vi "test-transform2d.vi"(8 "error in (no error)":errorcluster) -> (0 "error out":errorcluster, 3 "All PASSED":bool)   [LabVIEW 2019]
uses:
  <vilib>/Rock Robotics/WPI/ThirdParty/JAS_Junk/TrajLib/Transform2d_Create_PosePose.vi
  <vilib>/Rock Robotics/WPI/ThirdParty/JAS_Junk/TrajLib/Pose2d_New.vi
  <vilib>/Rock Robotics/WPI/ThirdParty/JAS_Junk/TrajLib/Pose2d_TransformBy.vi
  <vilib>/Rock Robotics/WPI/ThirdParty/JAS_Junk/TrajLib/Translation2d_Equals.vi
  <vilib>/Rock Robotics/WPI/ThirdParty/JAS_Junk/TrajLib/Rotation2d_Equals.vi
  <vilib>/Rock Robotics/WPI/ThirdParty/JAS_Junk/TrajLib/Translation2d_UnaryMinus.vi
  <vilib>/Rock Robotics/WPI/ThirdParty/JAS_Junk/TrajLib/Rotation2d_UnaryMinus.vi
  <vilib>/Rock Robotics/WPI/ThirdParty/JAS_Junk/TrajLib/Translation2d_RotateBy.vi
  <vilib>/Rock Robotics/WPI/ThirdParty/JAS_Junk/TrajLib/Translation2d_Minus.vi
  <vilib>/Rock Robotics/WPI/ThirdParty/JAS_Junk/TrajLib/Rotation2d_Minus.vi
  <vilib>/Rock Robotics/WPI/ThirdParty/JAS_Junk/TrajLib/Translation2d_Plus.vi
  <vilib>/Rock Robotics/WPI/ThirdParty/JAS_Junk/TrajLib/Rotation2d_Plus.vi
  <vilib>/Rock Robotics/WPI/ThirdParty/JAS_Junk/TrajLib/Util_CalcDist.vi
  <vilib>/Rock Robotics/WPI/ThirdParty/JAS_Junk/TrajLib/Rotation2d_RotateBy.vi
  <vilib>/Rock Robotics/WPI/ThirdParty/JAS_Junk/TrajLib/Rotation2d_CreateXY.vi
  <vilib>/Rock Robotics/WPI/ThirdParty/JAS_Junk/TrajLib/Trajectory_Library.lvlib
panel:
  out "Test 2 Passed":bool
  out "T1 Passed":bool
  out "T5 - ANG = 43 Deg":dbl
  out "T5 - Y2 = 4.4":dbl
  out "T5 - X2= -3.33":dbl
  out "T5 - Y = 4.4":dbl
  out "T5 - X = -3.33":dbl
  # "Transform2D Test  --- NOT DONE"
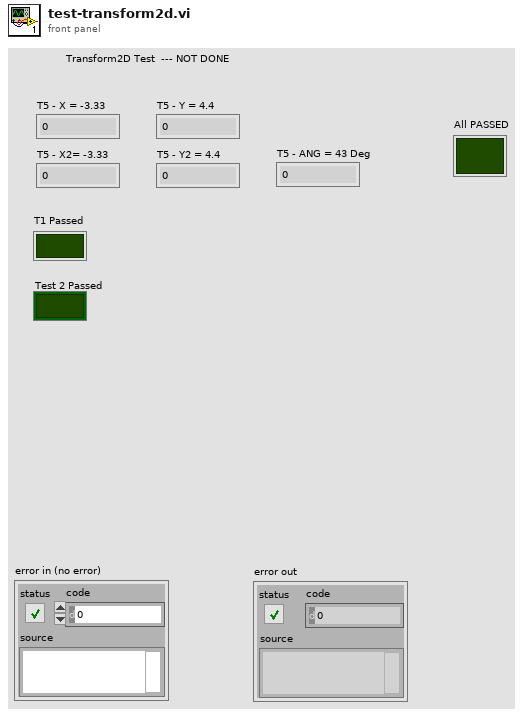
[diagram p1: front panel]
types:
  T1 = typedef "Trajectory_Library.lvlib/TRANSLATION2D.ctl" = cluster{"X":dbl, "Y":dbl}
  T2 = typedef "Trajectory_Library.lvlib/ROTATION2D.ctl" = cluster{"VALUE":dbl, "COS":dbl, "SIN":dbl}
  T3 = typedef "Trajectory_Library.lvlib/TRANSFORM2D.ctl" = cluster{"TRANSLATION":T1, "ROTATION":T2}
  T4 = typedef "Trajectory_Library.lvlib/POSE2D.ctl" = cluster{"TRANSLATION":T1, "ROTATION":T2}
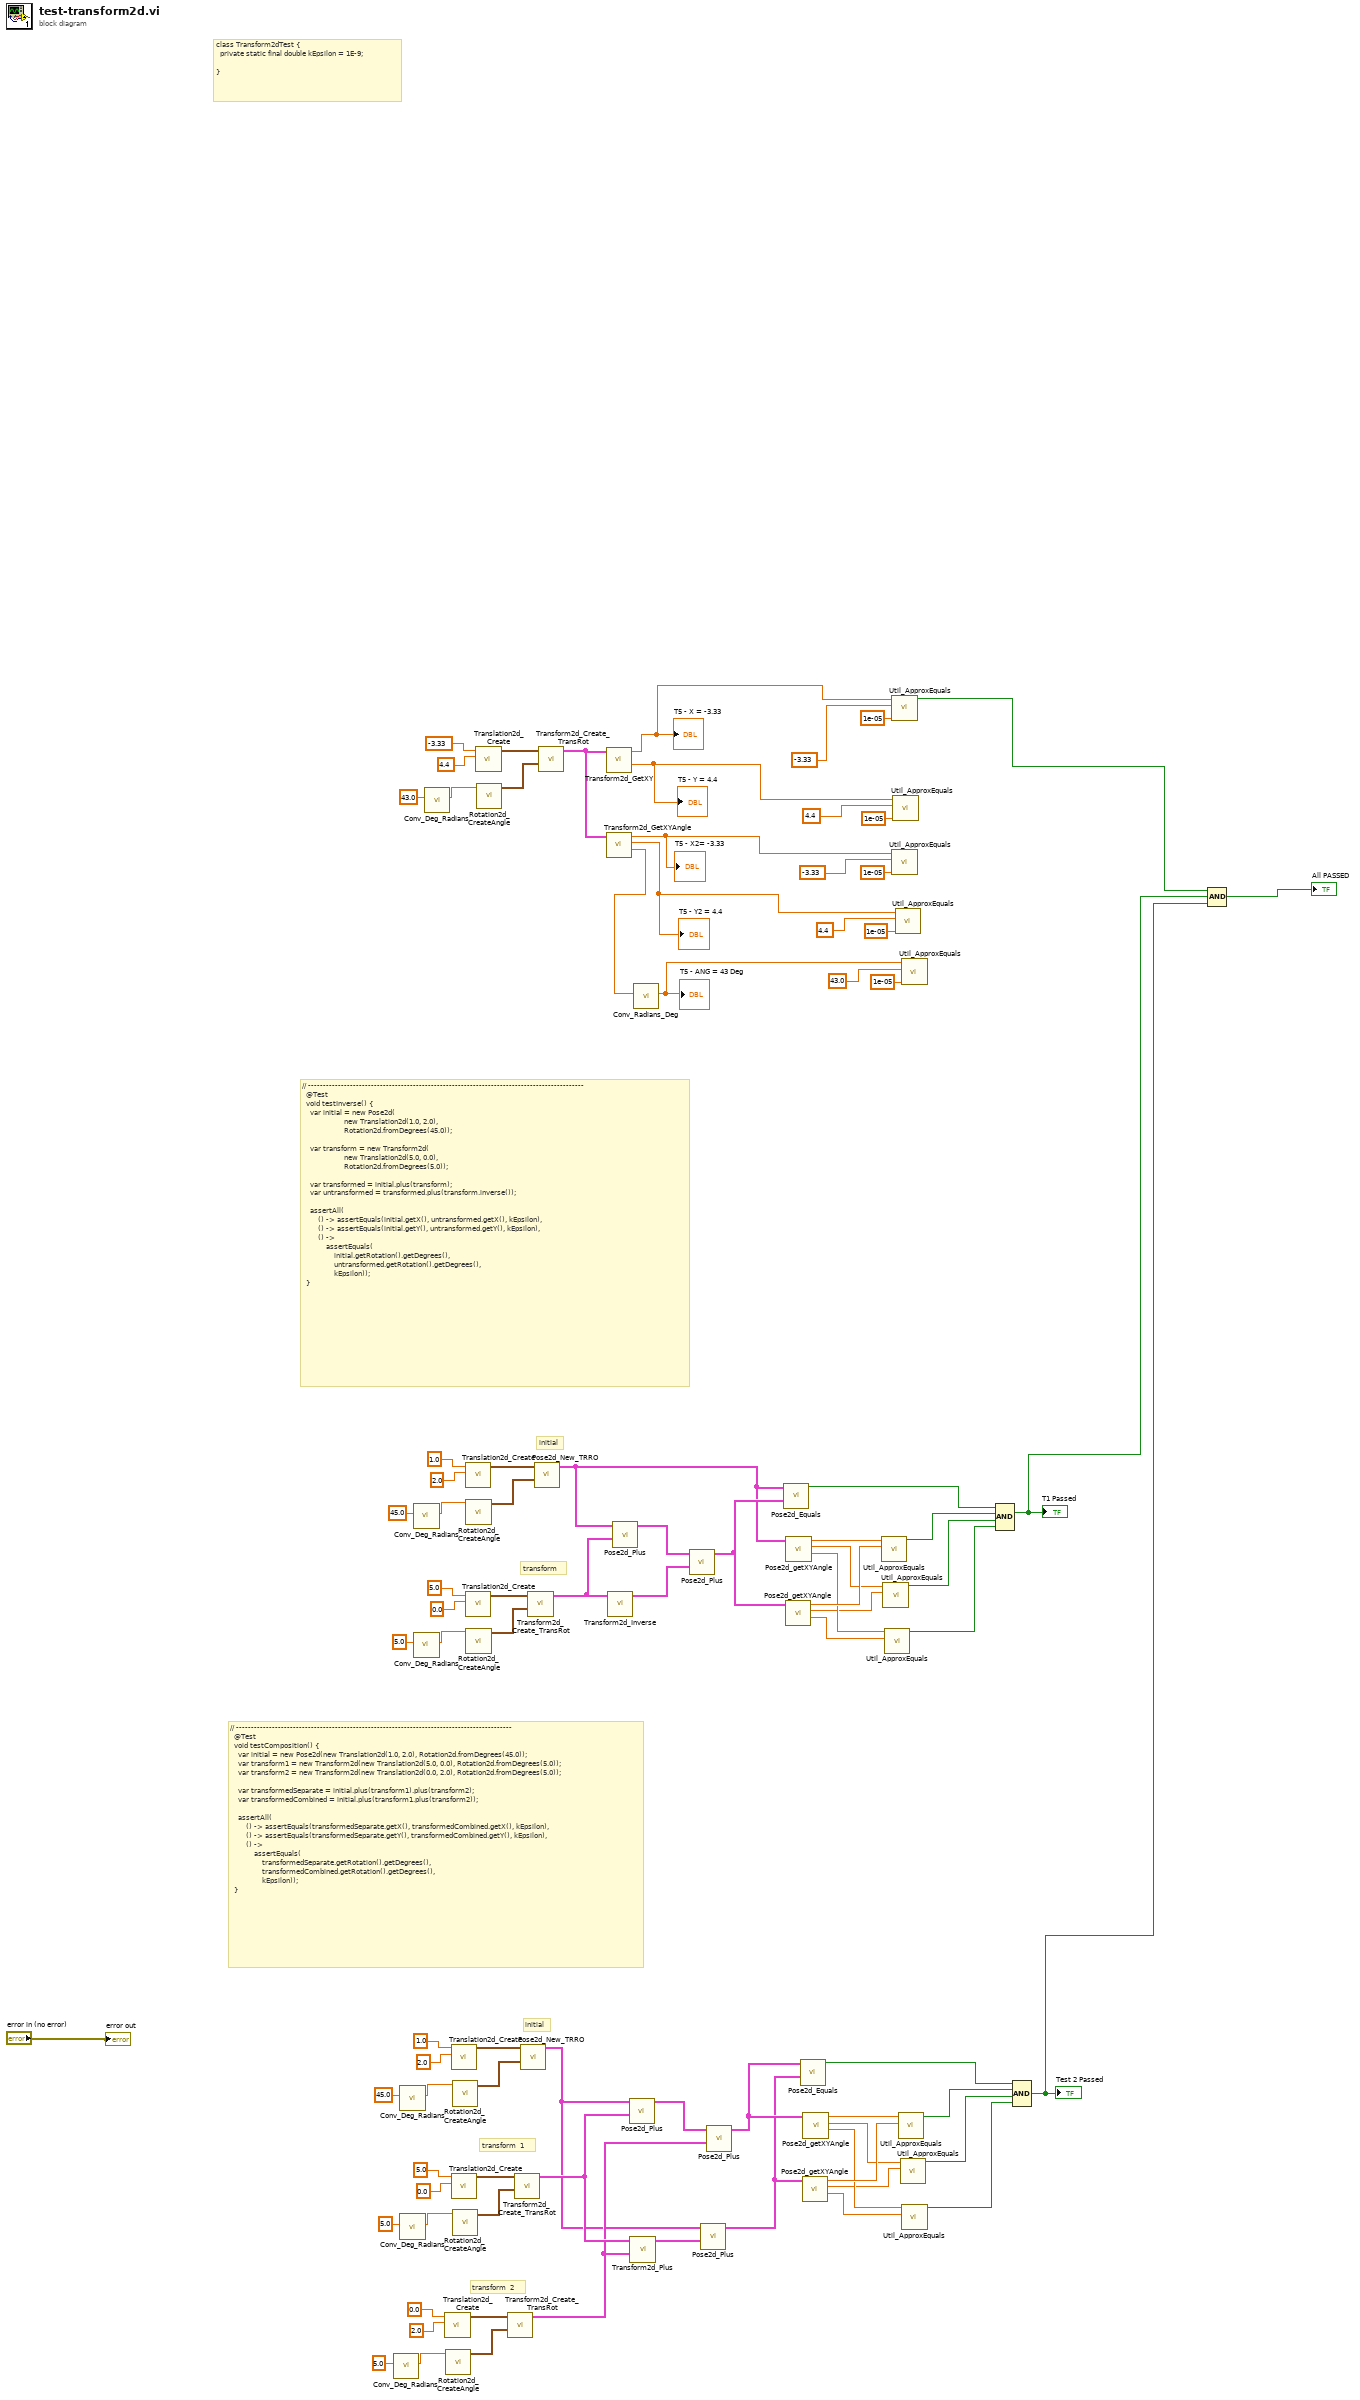
[diagram p0: block diagram]
diagram:
  # "transform  2"
  # "transform  1"
  # "initial"
  # "transform"
  # "initial"
  # "// --------------------------------------------------------------------------------------------\n  @Test\n  void testComposition() {\n    var initial = new Pose2d(new Translation2d(1.0, 2.0), Rotation2d.fromDegrees(45.0));\n    var transform1 = new Transform2d(new Translation2d(5.0, 0.0), Rotation2d.fromDegrees(5.0));\n    var transform2 = new Transform2d(new Translation2d(0.0, 2.0), Rotation2d.fromDegrees(5.0));\n\n    var transformedSeparate = initial.plus(transform1).plus(transform2);\n    var transformedCombined = initial.plus(transform1.plus(transform2));\n\n    assertAll(\n        () -> assertEquals(transformedSeparate.getX(), transformedCombined.getX(), kEpsilon),\n        () -> assertEquals(transformedSeparate.getY(), transformedCombined.getY(), kEpsilon),\n        () ->\n            assertEquals(\n                transformedSeparate.getRotation().getDegrees(),\n                transformedCombined.getRotation().getDegrees(),\n                kEpsilon));\n  }"
  # "// --------------------------------------------------------------------------------------------\n  @Test\n  void testInverse() {\n    var initial = new Pose2d(\n                     new Translation2d(1.0, 2.0), \n                     Rotation2d.fromDegrees(45.0));\n\n    var transform = new Transform2d(\n                     new Translation2d(5.0, 0.0), \n                     Rotation2d.fromDegrees(5.0));\n\n    var transformed = initial.plus(transform);\n    var untransformed = transformed.plus(transform.inverse());\n\n    assertAll(\n        () -> assertEquals(initial.getX(), untransformed.getX(), kEpsilon),\n        () -> assertEquals(initial.getY(), untransformed.getY(), kEpsilon),\n        () ->\n            assertEquals(\n                initial.getRotation().getDegrees(),\n                untransformed.getRotation().getDegrees(),\n                kEpsilon));\n  }"
  # "class Transform2dTest {\n  private static final double kEpsilon = 1E-9;\n\n}"
  n1 = call <vilib>:"Conv_Deg_Radians.vi"("Degress"=5.0) -> ("Radians"=w11:dbl)  [unwired: 10 in]
  n2 = call <vilib>:"Conv_Deg_Radians.vi"("Degress"=45.0) -> ("Radians"=w34:dbl)  [unwired: 10 in]
  n3 = call <vilib>:"Conv_Deg_Radians.vi"("Degress"=5.0) -> ("Radians"=w30:dbl)  [unwired: 10 in]
  n4 = call <vilib>:"Conv_Deg_Radians.vi"("Degress"=45.0) -> ("Radians"=w61:dbl)  [unwired: 10 in]
  n5 = call <vilib>:"Conv_Deg_Radians.vi"("Degress"=5.0) -> ("Radians"=w57:dbl)  [unwired: 10 in]
  n6 = call <vilib>:"Conv_Deg_Radians.vi"("Degress"=43.0) -> ("Radians"=w87:dbl)  [unwired: 10 in]
  n7 = call <vilib>:"Translation2d_Create.vi"("Y"=2.0, "X"=0.0) -> ("TRANSLATION"=w10:T1)  [unwired: 9 in]
  n8 = call <vilib>:"Rotation2d_CreateAngle.vi"("Angle"=w11) -> ("ROTATION"=w9:T2)  [unwired: 10 in]
  n9 = call <vilib>:"Translation2d_Create.vi"("Y"=2.0, "X"=1.0) -> ("TRANSLATION"=w27:T1)  [unwired: 9 in]
  n10 = call <vilib>:"Translation2d_Create.vi"("Y"=0.0, "X"=5.0) -> ("TRANSLATION"=w29:T1)  [unwired: 9 in]
  n11 = call <vilib>:"Rotation2d_CreateAngle.vi"("Angle"=w34) -> ("ROTATION"=w26:T2)  [unwired: 10 in]
  n12 = call <vilib>:"Rotation2d_CreateAngle.vi"("Angle"=w30) -> ("ROTATION"=w28:T2)  [unwired: 10 in]
  n13 = call <vilib>:"Translation2d_Create.vi"("Y"=2.0, "X"=1.0) -> ("TRANSLATION"=w54:T1)  [unwired: 9 in]
  n14 = call <vilib>:"Translation2d_Create.vi"("Y"=0.0, "X"=5.0) -> ("TRANSLATION"=w56:T1)  [unwired: 9 in]
  n15 = call <vilib>:"Rotation2d_CreateAngle.vi"("Angle"=w61) -> ("ROTATION"=w53:T2)  [unwired: 10 in]
  n16 = call <vilib>:"Rotation2d_CreateAngle.vi"("Angle"=w57) -> ("ROTATION"=w55:T2)  [unwired: 10 in]
  n17 = call <vilib>:"Translation2d_Create.vi"("Y"=4.4, "X"=-3.33) -> ("TRANSLATION"=w86:T1)  [unwired: 9 in]
  n18 = call <vilib>:"Rotation2d_CreateAngle.vi"("Angle"=w87) -> ("ROTATION"=w85:T2)  [unwired: 10 in]
  n19 = call <vilib>:"Transform2d_Create_TransRot.vi"("ROTATION"=w9, "TRANSLATION"=w10) -> ("TRANSFORM"=w7:T3)  [unwired: 9 in]
  n20 = call <vilib>:"Transform2d_Create_TransRot.vi"("ROTATION"=w28, "TRANSLATION"=w29) -> ("TRANSFORM"=w8:T3)  [unwired: 9 in]
  n21 = call <vilib>:"Pose2d_New_TRRO.vi"("ROTATION"=w26, "TRANSLATION"=w27) -> ("outPOSE"=w5:T4)  [unwired: 9 in]
  n22 = call <vilib>:"Transform2d_Create_TransRot.vi"("ROTATION"=w55, "TRANSLATION"=w56) -> ("TRANSFORM"=w51:T3)  [unwired: 9 in]
  n23 = call <vilib>:"Pose2d_New_TRRO.vi"("ROTATION"=w53, "TRANSLATION"=w54) -> ("outPOSE"=w48:T4)  [unwired: 9 in]
  n24 = call <vilib>:"Transform2d_Create_TransRot.vi"("ROTATION"=w85, "TRANSLATION"=w86) -> ("TRANSFORM"=w84:T3)  [unwired: 9 in]
  n25 = call <vilib>:"Transform2d_GetXY.vi"("inTRANSFORM"=w84) -> ("Y"=w73:dbl, "X"=w81:dbl)  [unwired: 9 in]
  "T5 - X = -3.33" <- w81
  "T5 - Y = 4.4" <- w73
  n26 = call <vilib>:"Transform2d_GetXYAngle.vi"("inTRANSFORM"=w84) -> ("Angle"=w83:dbl, "Y"=w69:dbl, "X"=w71:dbl)  [unwired: 8 in]
  "T5 - X2= -3.33" <- w71
  "T5 - Y2 = 4.4" <- w69
  n27 = call <vilib>:"Transform2d_Inverse.vi"("inTRANSFORM"=w51) -> ("TRANSFORM"=w50:T3)  [unwired: 10 in]
  n28 = call <vilib>:"Pose2d_Plus.vi"("other TRANSFORM"=w51, "in POSE"=w48) -> ("out POSE"=w52:T4)  [unwired: 9 in]
  n29 = call <vilib>:"Pose2d_Plus.vi"("other TRANSFORM"=w8, "in POSE"=w5) -> ("out POSE"=w25:T4)  [unwired: 9 in]
  n30 = call <vilib>:"Transform2d_Plus.vi"("otherTRANSFORM"=w7, "inTRANSFORM"=w8) -> ("TRANSFORM"=w6:T3)  [unwired: 9 in]
  n31 = call <vilib>:"Conv_Radians_Deg.vi"("Radians"=w83) -> ("Degrees"=w67:dbl)  [unwired: 10 in]
  "T5 - ANG = 43 Deg" <- w67
  n32 = call <vilib>:"Pose2d_Plus.vi"("other TRANSFORM"=w50, "in POSE"=w52) -> ("out POSE"=w49:T4)  [unwired: 9 in]
  n33 = call <vilib>:"Pose2d_Plus.vi"("other TRANSFORM"=w6, "in POSE"=w5) -> ("out POSE"=w3:T4)  [unwired: 9 in]
  n34 = call <vilib>:"Pose2d_Plus.vi"("other TRANSFORM"=w7, "in POSE"=w25) -> ("out POSE"=w4:T4)  [unwired: 9 in]
  n35 = call <vilib>:"Pose2d_Equals.vi"("other POSE"=w49, "in POSE"=w48) -> ("Equals"=w44:bool)  [unwired: 9 in]
  n36 = call <vilib>:"Pose2d_getXYAngle.vi"("in POSE"=w49) -> ("Angle"=w39:dbl, "Y"=w40:dbl, "X"=w46:dbl)  [unwired: 8 in]
  n37 = call <vilib>:"Pose2d_getXYAngle.vi"("in POSE"=w48) -> ("Angle"=w41:dbl, "Y"=w45:dbl, "X"=w47:dbl)  [unwired: 8 in]
  n38 = call <vilib>:"Pose2d_Equals.vi"("other POSE"=w3, "in POSE"=w4) -> ("Equals"=w21:bool)  [unwired: 9 in]
  n39 = call <vilib>:"Pose2d_getXYAngle.vi"("in POSE"=w3) -> ("Angle"=w16:dbl, "Y"=w17:dbl, "X"=w23:dbl)  [unwired: 8 in]
  n40 = call <vilib>:"Pose2d_getXYAngle.vi"("in POSE"=w4) -> ("Angle"=w18:dbl, "Y"=w22:dbl, "X"=w24:dbl)  [unwired: 8 in]
  n41 = call <vilib>:"Util_ApproxEquals.vi"("Value 2"=w46, "Value 1"=w47) -> ("ApproxEquals"=w43:bool)  [unwired: 9 in]
  n42 = call <vilib>:"Util_ApproxEquals.vi"("Value 2"=w40, "Value 1"=w45) -> ("ApproxEquals"=w42:bool)  [unwired: 9 in]
  n43 = call <vilib>:"Util_ApproxEquals.vi"("Value 2"=w39, "Value 1"=w41) -> ("ApproxEquals"=w38:bool)  [unwired: 9 in]
  n44 = call <vilib>:"Util_ApproxEquals.vi"("Tolerance"=1e-05, "Value 2"=-3.33 ("y"), "Value 1"=w81) -> ("ApproxEquals"=w78:bool)  [unwired: 8 in]
  n45 = call <vilib>:"Util_ApproxEquals.vi"("Tolerance"=1e-05, "Value 2"=-3.33 ("y"), "Value 1"=w71) -> ()  [unwired: 8 in, 1 out]
  n46 = call <vilib>:"Util_ApproxEquals.vi"("Tolerance"=1e-05, "Value 2"=4.4 ("y"), "Value 1"=w73) -> ()  [unwired: 8 in, 1 out]
  n47 = call <vilib>:"Util_ApproxEquals.vi"("Tolerance"=1e-05, "Value 2"=4.4 ("y"), "Value 1"=w69) -> ()  [unwired: 8 in, 1 out]
  n48 = call <vilib>:"Util_ApproxEquals.vi"("Value 2"=w23, "Value 1"=w24) -> ("ApproxEquals"=w20:bool)  [unwired: 9 in]
  n49 = call <vilib>:"Util_ApproxEquals.vi"("Value 2"=w17, "Value 1"=w22) -> ("ApproxEquals"=w19:bool)  [unwired: 9 in]
  n50 = call <vilib>:"Util_ApproxEquals.vi"("Tolerance"=1e-05, "Value 2"=43.0 ("y"), "Value 1"=w67) -> ()  [unwired: 8 in, 1 out]
  n51 = call <vilib>:"Util_ApproxEquals.vi"("Value 2"=w16, "Value 1"=w18) -> ("ApproxEquals"=w15:bool)  [unwired: 9 in]
  n52 = Compound Arithmetic op=AND(w44, w43, w42, w38) -> (w2:bool)
  "T1 Passed" <- w2
  n53 = Compound Arithmetic op=AND(w21, w20, w19, w15) -> (w1:bool)
  "Test 2 Passed" <- w1
  n54 = Compound Arithmetic op=AND(w78, w2, w1) -> (→"All PASSED":bool)
  "error out" <- "error in (no error)"
